vi "Gain.vi"(11 "Test Case In":refnum<class "Test.Camera.lvclass">) -> (0 "error out":errorcluster, 3 "Test Case Out":refnum<class "Test.Camera.lvclass">)   [LabVIEW 2020, in "Test.Camera.lvclass"]
uses:
  Test.Camera.lvclass
  Test.Camera.lvclass/Test.Camera.ctl
  <vilib>/Astemes/LUnit/Test Case.lvclass
  g_industrial_cam/Camera/Camera.lvclass
  c3e2611f-c54f-4219-a549-b8da21c7f085.vi
  C:/Program Files (x86)/National Instruments/LabVIEW 2020/vi.lib/Astemes/LUnit/Test Case.lvclass
  C:/Program Files (x86)/National Instruments/LabVIEW 2020/vi.lib/Astemes/LUnit/LUnit Runnable.lvclass
  C:/serenial/lib/g-industrial-camera/LabVIEW/tests/Test.Camera/Test.Camera.lvclass
  65a9066d-3369-419b-a362-ec50a561b226.vi
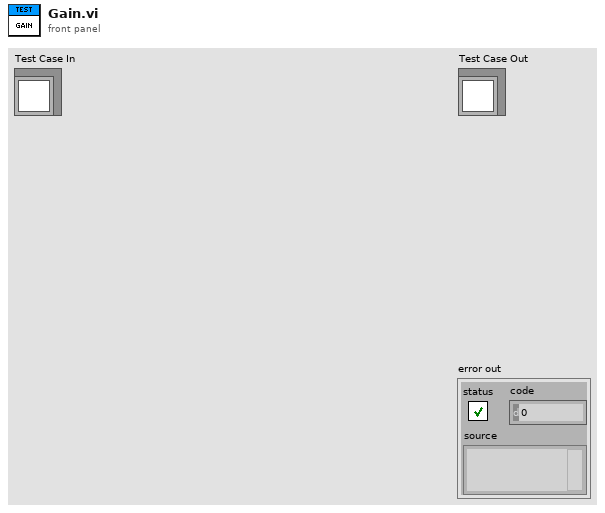
[diagram p1: front panel]
types:
  T1 = typedef "Camera.lvclass/Auto Mode.ctl" = enum8{"Off", "Once", "Continuous"}
  T2 = typedef "Camera.lvclass/Representation.ctl" = enum8{"Undefined", "Linear", "Logarithmic", "Boolean", "Pure Number", "Hex Number", "IP Address", "MAC Address"}
  T3 = cluster{"Representation":T2, "Min":dbl, "Max":dbl, "Mode":T1, "Avaliable":bool, "Gain":dbl, "Available Gains":string[]}
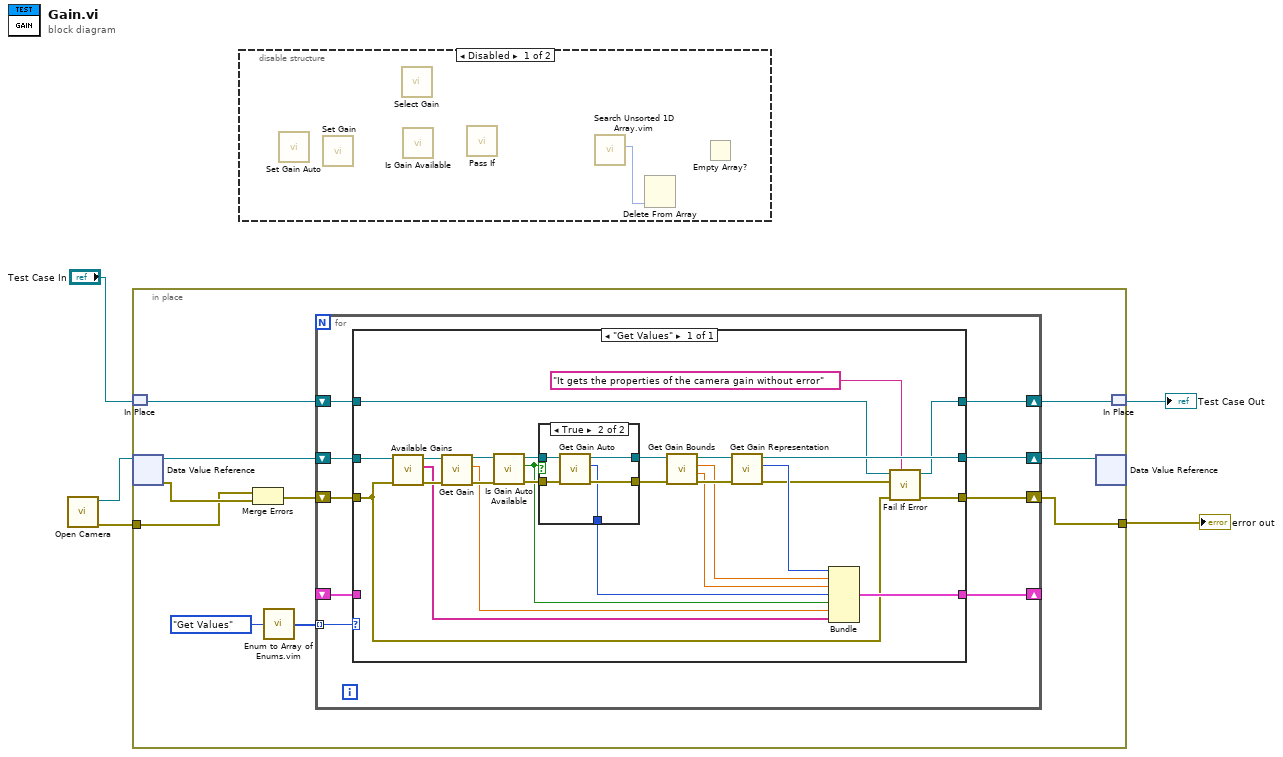
[diagram p0: block diagram]
diagram:
  n1 = call "Open Camera.vi"() -> ("error out"=w5:errorcluster, "Camera"=w4:refnum<data-value>)  [unwired: 10 in]
  n2 = in-place {
    in-place-border: w5 -> [w7]
    in-place-border: [w6] -> w2
    n3 = in-place-match #1("Test Case In") -> (w10:refnum<class "Test.Camera.lvclass">)
    n4 = in-place-dvr #2(w4) -> (w14:refnum<class "Camera.lvclass">, w15:errorcluster)
    n5 = Merge Errors(w7, w15) -> (w13:errorcluster)
    n6 = call "Enum to Array of Enums.vim"("enum"=enum16{"Get Values"}."Get Values") -> ("array of enums"=w11:enum16{"Get Values"}[])
    n7 = for {
      tunnel: w11 -> [w22] mode=indexing
      shift-right: [w21] -> w8
      shift-left: w14 -> [w24]
      shift-right: [w20] -> _
      shift-left: _ -> [w19]
      shift-right: [w17] -> w9
      shift-left: w10 -> [w18]
      shift-right: [w16] -> w6
      shift-left: w13 -> [w23]
      n8 = case shown="\"Get Values\"" w22 {
        tunnel: w24 -> [w50]
        tunnel: w23 -> [w28]
        tunnel: [w32] -> w21
        tunnel: [w31] -> w20
        tunnel: w19 -> [_]
        tunnel: w18 -> [w30]
        tunnel: [w29] -> w17
        tunnel: [w25] -> w16
        frame "Get Values" {
          n9 = call "Available Gains.vi"("error in (no error)"=w28, "Camera in"=w50) -> ("error out"=w47:errorcluster, "Available Gains"=w39:string[], "Camera"=w49:refnum<class "Camera.lvclass">)  [unwired: 7 in]
          n10 = call "Get Gain.vi"("error in (no error)"=w47, "Camera in"=w49) -> ("error out"=w46:errorcluster, "Gain"=w38:dbl, "Camera"=w48:refnum<class "Camera.lvclass">)  [unwired: 7 in]
          n11 = call "Is Gain Auto Available.vi"("error in (no error)"=w46, "Camera in"=w48) -> ("error out"=w45:errorcluster, "Avaliable"=w37:bool, "Camera"=w44:refnum<class "Camera.lvclass">)  [unwired: 7 in]
          n12 = case shown="True" w37 {
            tunnel: w45 -> [w51 w57]
            tunnel: w44 -> [w52 w56]
            tunnel: [w52 w55] -> w42
            tunnel: [w51 w54] -> w43
            tunnel: [_ w53] -> w36
            frame False {
            }
            frame True {
              n13 = call "Get Gain Auto.vi"("error in (no error)"=w57, "Camera in"=w56) -> ("error out"=w54:errorcluster, "Mode"=w53:T1, "Camera"=w55:refnum<class "Camera.lvclass">)  [unwired: 7 in]
            }
          }
          n14 = call "Get Gain Bounds.vi"("error in (no error)"=w43, "Camera in"=w42) -> ("error out"=w41:errorcluster, "Max"=w35:dbl, "Min"=w34:dbl, "Camera"=w40:refnum<class "Camera.lvclass">)  [unwired: 6 in]
          n15 = call "Get Gain Representation.vi"("error in (no error)"=w41, "Camera in"=w40) -> ("error out"=w27:errorcluster, "Representation"=w33:T2, "Camera"=w32:refnum<class "Camera.lvclass">)  [unwired: 7 in]
          n16 = Bundle("Representation"=w33, "Min"=w34, "Max"=w35, "Mode"=w36, "Avaliable"=w37, "Gain"=w38, "Available Gains"=w39) -> (w31:T3)  [unwired: 1 in]
          n17 = call <vilib>:"Fail If Error.vi"("Description"="It gets the properties of the camera gain without error", "error in (no error)"=w28, "Assert error"=w27, "LUnit Test Case In"=w30) -> ("error out"=w25:errorcluster, "LUnit Test Case Out"=w29:refnum<class "Test.Camera.lvclass">)  [unwired: 6 in]
        }
      }
    }
    n18 = in-place-dvr #2(w8) -> ()  [unwired: 2 out]
    n19 = in-place-match #1(w9) -> (→"Test Case Out":refnum<class "Test.Camera.lvclass">)
  }
  "error out" <- w2
  n20 = disable-structure shown="Disabled" {
    frame Disabled {
      n21 = call "Set Gain Auto.vi"() -> ()  [unwired: 10 in, 2 out]
      n22 = call "Set Gain.vi"() -> ()  [unwired: 10 in, 2 out]
      n23 = call "Select Gain.vi"() -> ()  [unwired: 10 in, 2 out]
      n24 = call "Is Gain Available.vi"() -> ()  [unwired: 9 in, 3 out]
      n25 = call <vilib>:"Pass If.vi"() -> ()  [unwired: 10 in, 2 out]
      n26 = call "Search Unsorted 1D Array.vim"() -> ("index of element"=w58:i32)  [unwired: 11 in]
      n27 = Delete From Array(index=w58) -> ()  [unwired: 2 in, 2 out]
      n28 = Empty Array?() -> ()  [unwired: 1 in, 1 out]
    }
    frame Enabled {
    }
  }
